vi "close.vi"(8 "error in (no error)":errorcluster, 11 "Instrument in":refnum<class "Picomotor.lvclass">) -> (0 "error out":errorcluster)   [LabVIEW 2020, in "Picomotor.lvclass"]
uses:
  Picomotor.lvclass
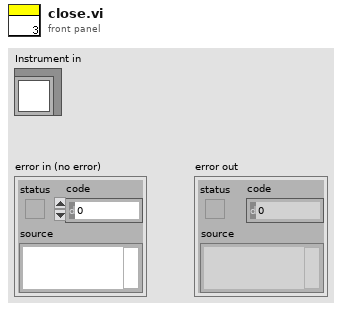
[diagram p1: front panel]
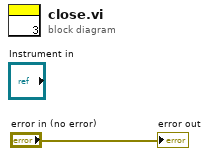
[diagram p0: block diagram]
diagram:
  "error out" <- "error in (no error)"
